vi "Joystick_Inputs_to_Commands.vi"(11 "Joystick Inputs":T4) -> (3 "All Commands":T1)   [LabVIEW 2012]
uses:
  Joystick_Inputs.ctl
  <vilib>/Rock Robotics/WPI/Joystick/WPI_JoystickButtonState.ctl
  All_Commands.ctl
  Cirular Shooter/circular_shooter_commands.ctl
  Climber/Climber_Commands.ctl
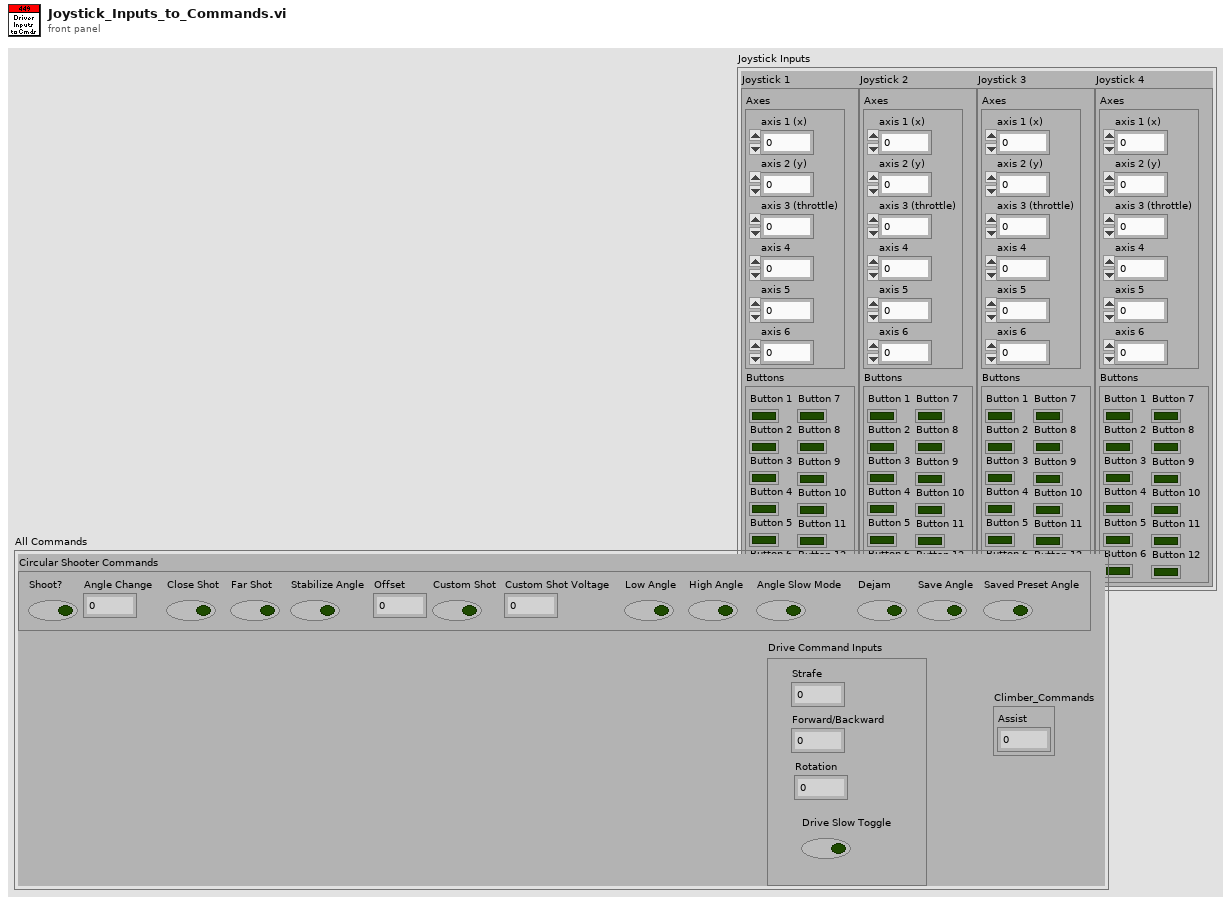
[diagram p1: front panel]
types:
  T1 = typedef "All_Commands.ctl" = cluster{"Circular Shooter Commands":T2, "Drive Command Inputs":cluster{"Strafe":dbl, "Forward/Backward":dbl, "Rotation":dbl, "Drive Slow Toggle":bool}, "Climber_Commands":T3}
  T2 = typedef "circular_shooter_commands.ctl" = cluster{"Shoot?":bool, "Angle Change":dbl, "Close Shot":bool, "Far Shot":bool, "Stabilize Angle ":bool, "Offset":dbl, "Custom Shot":bool, "Custom Shot Voltage":dbl, "Low Angle":bool, "High Angle":bool, "Angle Slow Mode":bool, "Dejam":bool, "Save Angle":bool, "Saved Preset Angle":bool}
  T3 = typedef "Climber_Commands.ctl" = cluster{"Assist":dbl}
  T4 = typedef "Joystick_Inputs.ctl" = cluster{"Joystick 1":cluster{"Axes":cluster{"axis 1 (x)":dbl, "axis 2 (y)":dbl, "axis 3 (throttle)":dbl, "axis 4":dbl, "axis 5":dbl, "axis 6":dbl}, "Buttons":T5}, "Joystick 2":cluster{"Axes":cluster{"axis 1 (x)":dbl, "axis 2 (y)":dbl, "axis 3 (throttle)":dbl, "axis 4":dbl, "axis 5":dbl, "axis 6":dbl}, "Buttons":T5}, "Joystick 3":cluster{"Axes":cluster{"axis 1 (x)":dbl, "axis 2 (y)":dbl, "axis 3 (throttle)":dbl, "axis 4":dbl, "axis 5":dbl, "axis 6":dbl}, "Buttons":T5}, "Joystick 4":cluster{"Axes":cluster{"axis 1 (x)":dbl, "axis 2 (y)":dbl, "axis 3 (throttle)":dbl, "axis 4":dbl, "axis 5":dbl, "axis 6":dbl}, "Buttons":T5}}
  T5 = typedef "WPI_JoystickButtonState.ctl" = cluster{"Button 1":bool, "Button 2":bool, "Button 3":bool, "Button 4":bool, "Button 5":bool, "Button 6":bool, "Button 7":bool, "Button 8":bool, "Button 9":bool, "Button 10":bool, "Button 11":bool, "Button 12":bool}
  T6 = cluster{"Strafe":dbl, "Forward/Backward":dbl, "Rotation":dbl, "Drive Slow":bool}
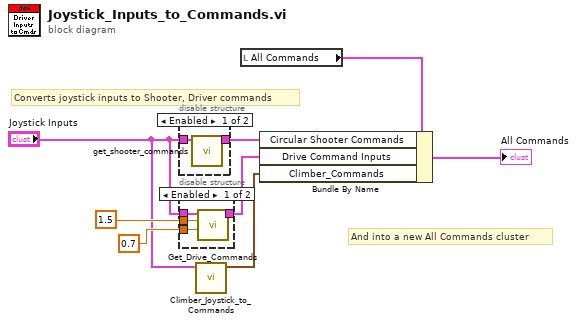
[diagram p0: block diagram]
diagram:
  # "And into a new All Commands cluster"
  # "Converts joystick inputs to Shooter, Driver commands"
  n1 = disable-structure shown="Enabled" {
    disable-tunnel: [w10 _] -> w8
    disable-tunnel: "Joystick Inputs" -> [w9 _]
    frame Enabled {
      n2 = call "get_shooter_commands.vi"("Driver Inputs"=w9) -> ("Circular Shooter Commands"=w10:T2)  [unwired: 10 in]
    }
    frame Disabled {
    }
  }
  n3 = disable-structure shown="Enabled" {
    disable-tunnel: "Joystick Inputs" -> [w14 _]
    disable-tunnel: [w13 _] -> w5
    disable-tunnel: 0.7 ("Rotation Multiplier") -> [w12 _]
    disable-tunnel: 1.5 -> [w11 _]
    frame Enabled {
      n4 = call "Get_Drive_Commands.vi"("Rotation Multiplier"=w12, "Strafe Multiplier"=w11, "Driver Inputs"=w14) -> ("Drive Command Inputs"=w13:T6)  [unwired: 8 in]
    }
    frame Disabled {
    }
  }
  n5 = call "Climber_Joystick_to_Commands.vi"("Driver Inputs"="Joystick Inputs") -> ("Climber_Commands"=w1:T3)  [unwired: 10 in]
  n6 = local read "All Commands"() -> (w6:T1)
  n7 = Bundle By Name(cluster=w6, "Circular Shooter Commands"=w8, "Drive Command Inputs"=w5, "Climber_Commands"=w1) -> (→"All Commands":T1)
